vi "alarm_what.vi"(2 "状态":string="状态", 3 "报警":string="报警") -> (0 "Alarm":string[](array[string]))   [LabVIEW 2015]
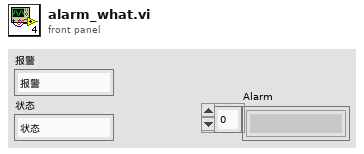
[diagram p1: front panel]
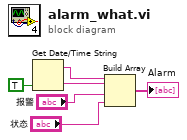
[diagram p0: block diagram]
diagram:
  n1 = Get Date/Time String(want seconds? (F)=TRUE ("需要秒？(F)")) -> (date string=w5:string, time string=w4:string)  [unwired: 2 in]
  n2 = Build Array(w5, w4, "报警", "状态") -> (→"Alarm":string[])
